vi "Read Element of Multpart_Form-Data.vi"(8 "error in (no error)":errorcluster, 10 "index":i32, 11 "Request in":refnum<class "Request.lvclass">) -> (0 "error out":errorcluster, 2 "Element":T1={"Name"="", "Value"="", "File"=path "", "Filename"="", "MIME type"="application/octet-stream"}, 3 "Request out":refnum<class "Request.lvclass">)   [LabVIEW 2020, in "Request.lvclass"]
uses:
  Request/Request.lvclass
  Request/Request.lvclass/Request.ctl
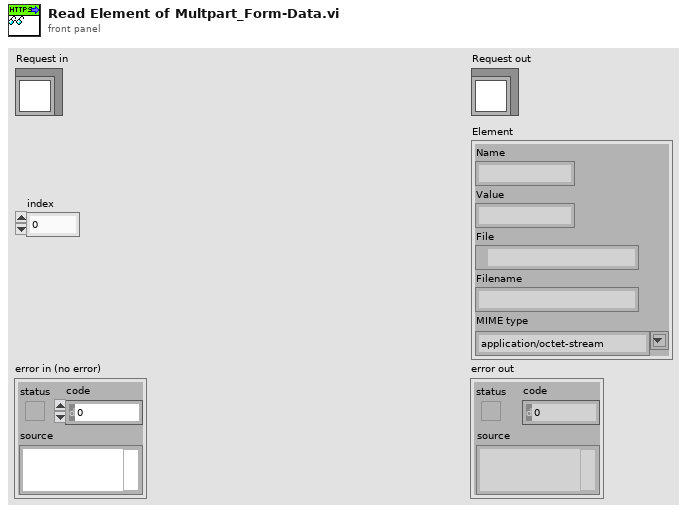
[diagram p1: front panel]
types:
  T1 = cluster{"Name":string, "Value":string, "File":path, "Filename":string, "MIME type":string}
  T2 = cluster{"Name":string, "Value":string, "File":path, "Filename":string, "MIME type":string}[]
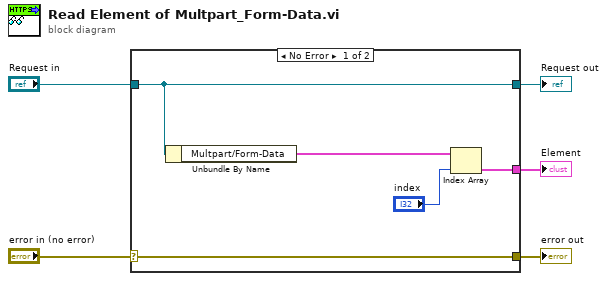
[diagram p0: block diagram]
diagram:
  n1 = case shown="No Error" "error in (no error)" {
    selector: "error in (no error)" -> [w10 w11]
    tunnel: [w10 w11] -> w4
    tunnel: [w9 w12] -> w2
    tunnel: "Request in" -> [w9 w12]
    tunnel: [w6 _] -> w1
    frame No Error {
      n2 = Unbundle By Name(w9) -> ("Multpart/Form-Data"=w8:T2)
      n3 = Index Array(array=w8, index="index") -> (element=w6:T1)
    }
    frame Error {
    }
  }
  "error out" <- w4
  "Request out" <- w2
  "Element" <- w1
